vi "WriteProduktID.vi"(8 "error in (no error)":errorcluster, 9 "ProductName":string, 10 "ProduktID":u32, 11 "BME_DG_Base in":refnum<class "BME_DG_Base.lvclass">) -> (0 "error out":errorcluster, 3 "BME_DG_Base out":refnum<class "BME_DG_Base.lvclass">)   [LabVIEW 2009, in "POLARIS BME DG.lvlib" / "BME_DG_Base.lvclass"]
uses:
  BME_DG_Base.lvclass
  BME_DG_Base.lvclass/BME_DG_Base.ctl
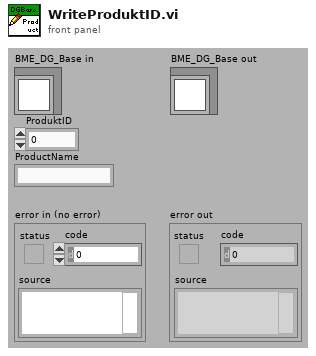
[diagram p1: front panel]
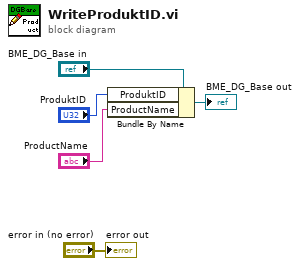
[diagram p0: block diagram]
diagram:
  n1 = Bundle By Name(cluster="BME_DG_Base in", "ProduktID"="ProduktID", "ProductName"="ProductName") -> (→"BME_DG_Base out":refnum<class "BME_DG_Base.lvclass">)
  "error out" <- "error in (no error)"
